vi "UI_AutoRefresh_Do.vi"(8 "error in (no error)":errorcluster, 9 "Parameters":T1={"Write TipStrips with details (T)"=TRUE, "Write Captions with UserLabels (T)"=TRUE, "Mode (ind only)"=enum."Indicators only", "Enable nested stream (T)"=TRUE}, 10 "Databox_sealed":refnum<class "Databox_sealed.lvclass">, 11 "SingleIndi in":refnum<class "SingleIndi.lvclass">) -> (0 "error out":errorcluster, 3 "SingleIndi out":refnum<class "SingleIndi.lvclass">)   [LabVIEW 2020, in "SingleIndi.lvlib" / "SingleIndi.lvclass"]
doc: "Enable nested stream : Permet le routage de la databox vers les nested UIA de l'acteur. On peut couper ce ruissellement si les nested n'ont pas besoin de databox pour optimiser le programme."
uses:
  SingleIndi.lvclass
  D:/Projets/IRSN/464 - IRSN - LEF/464-irsn-lef-hmi/support/UI_Actor.lvlibp/UI_Actor/UI_Actor.lvclass
  support/UI_Actor.lvlibp/UI_Actor/ctl_AR_Parameters.ctl
  support/UI_Actor.lvlibp/UI_Actor/ctl_AR_Mode.ctl
  support/Databox.lvlibp/Databox_sealed/Databox_sealed.lvclass
  support/UI_Actor.lvlibp/UI_Actor/UI_Elmt_Read(Label)-Strg.vi
  support/Databox.lvlibp/TypesTools/Config/Read Unit.vi
  support/UI_Actor.lvlibp/UI_Actor/UI_Elmt_Write(Label).vi
  D&C_SchemaBase/D&C_SchemaBase/D&C_SchemaBase.lvclass
  support/UI_Actor.lvlibp/UI_Actor/UI_Actor.lvclass
  D:/Projets/IRSN/464 - IRSN - LEF/464-irsn-lef-hmi/D&Cs/D&C_SchemaBase/D&C_SchemaBase/D&C_SchemaBase.lvclass
  D:/Projets/IRSN/464 - IRSN - LEF/464-irsn-lef-hmi/support/Actor Framework.lvlibp/1abvi3w/vi.lib/ActorFramework/Actor/Actor.lvclass
  D:/Projets/IRSN/464 - IRSN - LEF/464-irsn-lef-hmi/D&Cs/SingleIndi/SingleIndi/SingleIndi.lvclass
  support/Databox.lvlibp/TypesTools/Data/Data.lvclass
  support/Databox.lvlibp/TypesTools/Config/Config.lvclass
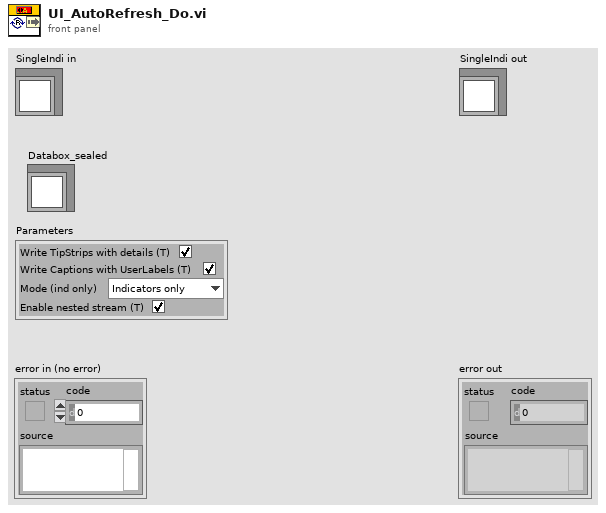
[diagram p1: front panel]
types:
  T1 = typedef "UI_Actor.lvlibp/UI_Actor.lvclass/ctl_AR_Parameters.ctl" = cluster{"Write TipStrips with details (T)":bool, "Write Captions with UserLabels (T)":bool, "Mode (ind only)":T2, "Enable nested stream (T)":bool}
  T2 = typedef "UI_Actor.lvlibp/UI_Actor.lvclass/ctl_AR_Mode.ctl" = enum16{"Controls only", "Indicators only", "All"}
  T3 = typedef "UI_Actor.lvlibp/UI_Actor.lvclass/ctl_InternalMapItem.ctl" = cluster{"Config":refnum<class "Config.lvclass">, "LatestData":refnum<class "Data.lvclass">}
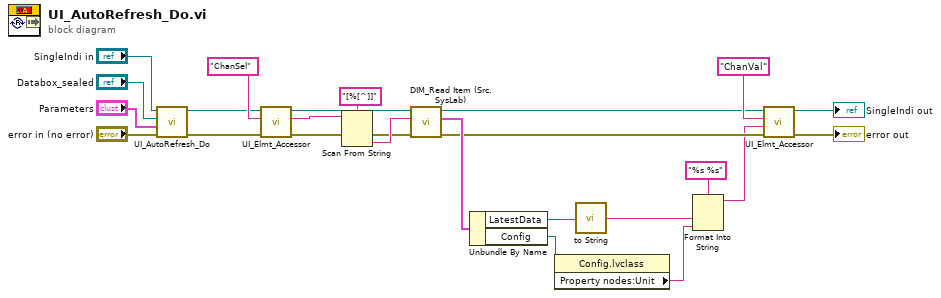
[diagram p0: block diagram]
diagram:
  n1 = call-parent "UI_AutoRefresh_Do.vi"("error in (no error)"="error in (no error)", "Parameters"="Parameters", "Databox_sealed"="Databox_sealed", "UI_Actor in"="SingleIndi in") -> ("error out"=w18:errorcluster, "UI_Actor out"=w19:refnum<class "SingleIndi.lvclass">)  [unwired: 6 in]
  n2 = call-poly "UI_Elmt_Accessor.vi"("error in (no error)"=w18, "Elmt Label"="ChanSel", "UI_Actor in"=w19) -> ("error out"=w2:errorcluster, "Value"=w3:string, "UI_Actor out"=w12:refnum<class "SingleIndi.lvclass">)  [unwired: 5 in, 1 out]
  n3 = Scan From String(format string="[%[^]]", input string=w3, error in=w2) -> (error out=w1:errorcluster, output 1=w4:string)  [unwired: 2 in, 2 out]
  n4 = call "DIM_Read Item (Src.SysLab).vi"("error in (no error)"=w1, "Sourcer.SysLabel"=w4, "UI_Actor in"=w12) -> ("error out"=w10:errorcluster, "DIM Item"=w15:T3, "UI_Actor out"=w11:refnum<class "SingleIndi.lvclass">)  [unwired: 5 in, 1 out]
  n5 = Unbundle By Name(w15) -> ("LatestData"=w14:refnum<class "Data.lvclass">, "Config"=w13:refnum<class "Config.lvclass">)
  n6 = property class="Config.lvclass"(reference=w13) -> ("Property nodes:Unit"=w8:string)  [unwired: 1 in, 2 out]
  n7 = call "to String.vi"("Data"=w14) -> ("String"=w6:string)
  n8 = Format Into String(format string="%s %s", w6, w8) -> (resulting string=w7:string)  [unwired: 2 in, 1 out]
  n9 = call-poly "UI_Elmt_Accessor.vi"("error in (no error)"=w10, "Value"=w7, "Elmt Label"="ChanVal", "UI_Actor in"=w11) -> ("error out"=→"error out":errorcluster, "UI_Actor out"=→"SingleIndi out":refnum<class "SingleIndi.lvclass">)  [unwired: 5 in, 1 out]
